vi "Length Encoded Integer.vi"(0 "Bytes in":u8[](array[numeric]), 11 "Start Index(0)":i32) -> (4 "Remaining Bytes out":u8[](array[numeric]), 6 "Integer Bytes":u8[](array[numeric]), 8 "Integer":u64, 15 "End Index":i32)   [LabVIEW 2014, in "hse-db.lvlib" / "MySQL (TCP).lvlib"]
uses:
  MySQL (TCP).lvlib
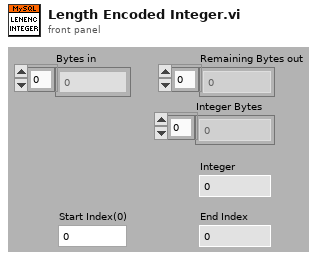
[diagram p1: front panel]
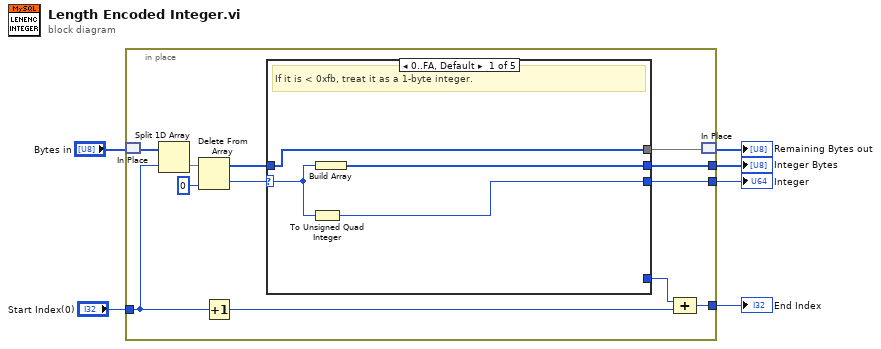
[diagram p0: block diagram]
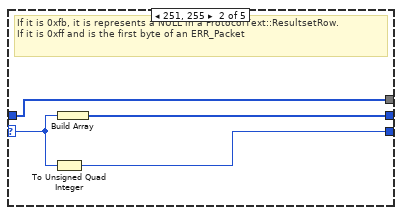
[diagram p2: hidden frame]
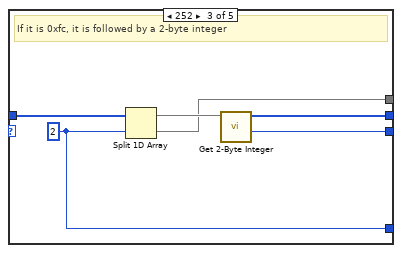
[diagram p3: hidden frame]
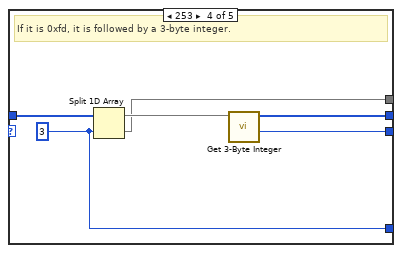
[diagram p4: hidden frame]
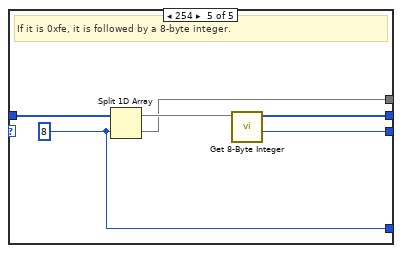
[diagram p5: hidden frame]
diagram:
  n1 = in-place {
    in-place-border: [w18] -> w6
    in-place-border: [w7] -> w5
    in-place-border: [w17] -> w4
    in-place-border: "Start Index(0)" -> [w15]
    n2 = in-place-match #1("Bytes in") -> (w16:u8[])
    n3 = Split 1D Array(array=w16, index=w15) -> (second subarray=w14:u8[])  [unwired: 1 out]
    n4 = Delete From Array(array=w14, index=0) -> (deleted portion=w13:u8, array with subset deleted=w11:u8[])  [unwired: 1 in]
    n5 = Increment(x=w15) -> (x+1=w9:i32)
    n6 = case shown="0..FA, Default" w13 {
      selector: w13 -> [w21 w25 _ _ _]
      tunnel: [w22 w26 w28 w33 w39] -> w18
      tunnel: w11 -> [w19 w23 w32 w38 w44]
      tunnel: [_ _ w29 w35 w41] -> w8
      tunnel: [w20 w24 w27 w34 w40] -> w17
      tunnel: [w19 w23 w30 w36 w42] -> w10
      frame 0..250, Default {
        # "If it is < 0xfb, treat it as a 1-byte integer."
        n7 = To Unsigned Quad Integer(1:w21) -> (0:w22:u64)
        n8 = Build Array(w21) -> (w20:u8[])
      }
      frame 251, 255 {
        # "If it is 0xfb, it is represents a NULL in a ProtocolText::ResultsetRow.\nIf it is 0xff and is the first byte of an ERR_Packet"
        n9 = To Unsigned Quad Integer(1:w25) -> (0:w26:u64)
        n10 = Build Array(w25) -> (w24:u8[])
      }
      frame 252 {
        w29 = 2 ("length")
        # "If it is 0xfc, it is followed by a 2-byte integer"
        n11 = Split 1D Array(array=w32, index=w29) -> (first subarray=w31:u8[], second subarray=w30:u8[])
        n12 = call "Get 2-Byte Integer.vi"("Bytes in"=w31) -> ("2-Byte Integer"=w28:u64, "Bytes out"=w27:u8[])  [unwired: 9 in]
      }
      frame 253 {
        w35 = 3 ("length")
        # "If it is 0xfd, it is followed by a 3-byte integer."
        n13 = Split 1D Array(array=w38, index=w35) -> (first subarray=w37:u8[], second subarray=w36:u8[])
        n14 = call "Get 3-Byte Integer.vi"("Bytes in"=w37) -> ("3-Byte Integer"=w33:u64, "Bytes out"=w34:u8[])  [unwired: 9 in]
      }
      frame 254 {
        w41 = 8 ("y")
        # "If it is 0xfe, it is followed by a 8-byte integer."
        n15 = Split 1D Array(array=w44, index=w41) -> (first subarray=w43:u8[], second subarray=w42:u8[])
        n16 = call "Get 8-Byte Integer.vi"("Bytes in"=w43) -> ("8-Byte Integer"=w39:u64, "Bytes out"=w40:u8[])  [unwired: 9 in]
      }
    }
    n17 = Compound Arithmetic op=ADD(w8, w9) -> (w7:i32)
    n18 = in-place-match #1(w10) -> (→"Remaining Bytes out":u8[])
  }
  "Integer" <- w6
  "End Index" <- w5
  "Integer Bytes" <- w4
